vi "AudioTest, Audio Test Util, Manager.vi"(8 "error in (no error)":errorcluster, 11 "Config Folder":path=path "C:/MTE/Audio Test/Config") -> (0 "Error Out":errorcluster, 1 "Audio Test Result Path":path, 2 "Audio Test App Path":path, 3 "Meas":T1 {"Status" items=["LOG", "PASS", "FAIL", "ERROR"]})   [LabVIEW 2018]
uses:
  Common/Utils/Results/Result.Measurement Item.ctl
  Common/Utils/Results/Result.Measurement and Attribute Item Status.ctl
  Common/Utils/Cmd Exe/CmdConsole/CmdConsole.lvclass
  <vilib>/KATE/Files/File Utils.lvlib
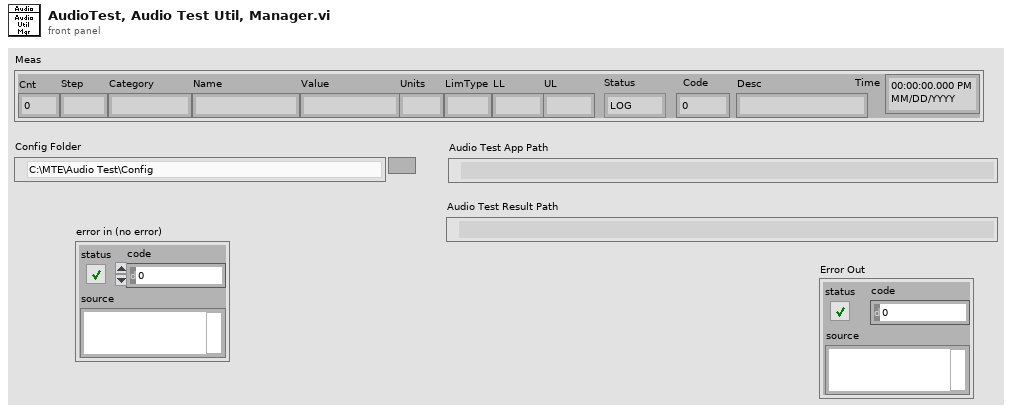
[diagram p1: front panel]
types:
  T1 = typedef "Result.Measurement Item.ctl" = cluster{"Cnt":i32, "Step":string, "Category":string, "Name":string, "Value":string, "Units":string, "LimType":string, "LL":string, "UL":string, "Status":T2, "Code":i32, "Desc":string, "Time":timestamp}
  T2 = typedef "Result.Measurement and Attribute Item Status.ctl" = i32
  T3 = enum32{"invalid app kind", "Development System", "Run Time System", "Student Edition", "Embedded LabVIEW", "Evaluation", "Custom"}
  T4 = cluster{"CmdConsole":refnum<class "CmdConsole.lvclass">, "OutDir":path, "Meas":T1}
  T5 = typedef "FunctTest.Result State.ctl" = enum32{"NoTest", "PASS", "FAIL"}
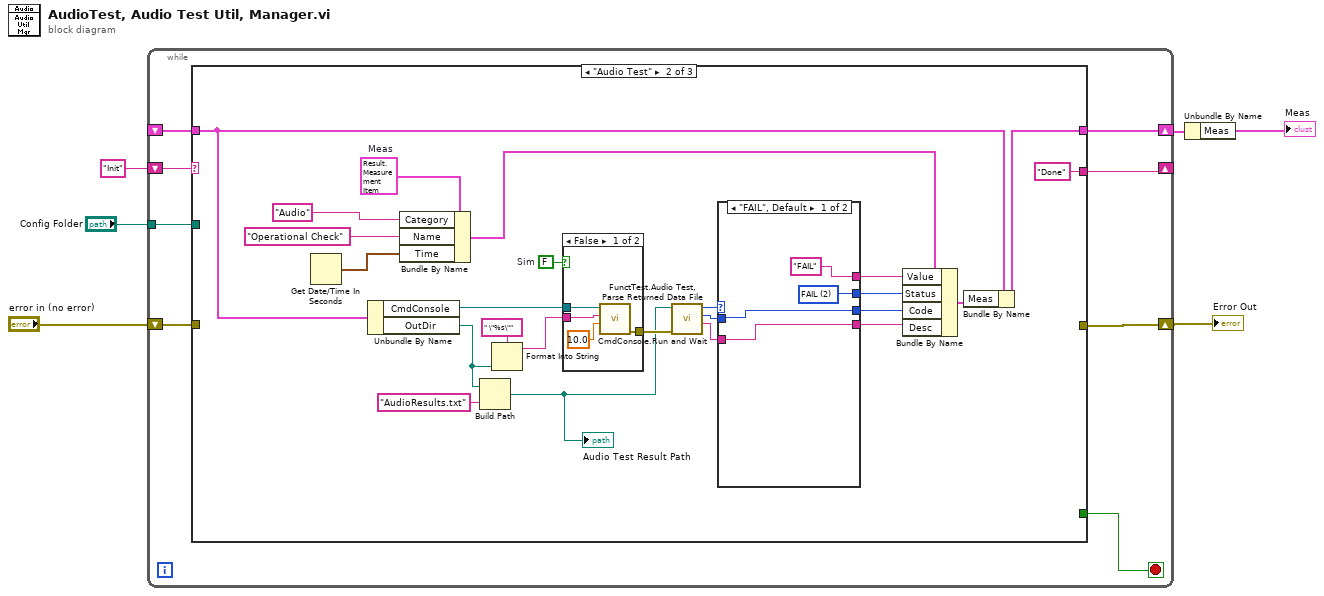
[diagram p0: block diagram]
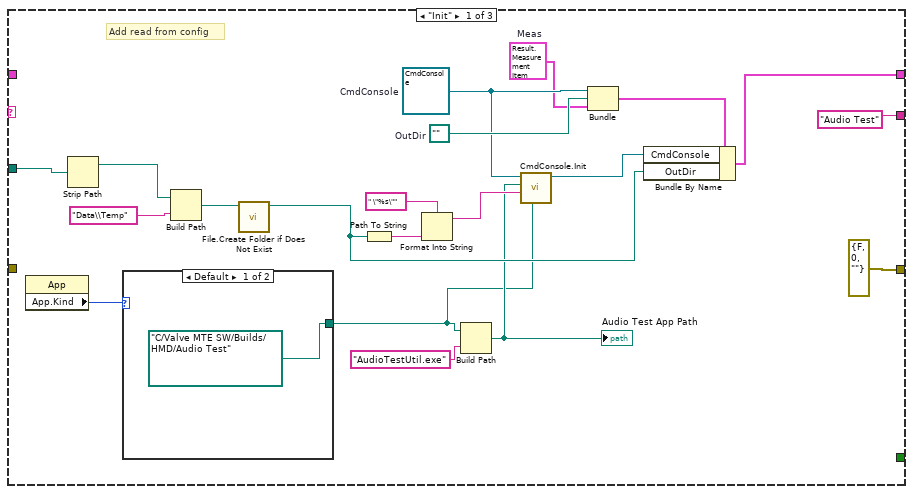
[diagram p2: hidden frame]
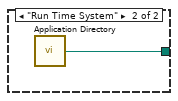
[diagram p3: hidden frame]
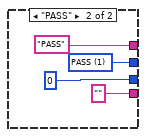
[diagram p4: hidden frame]
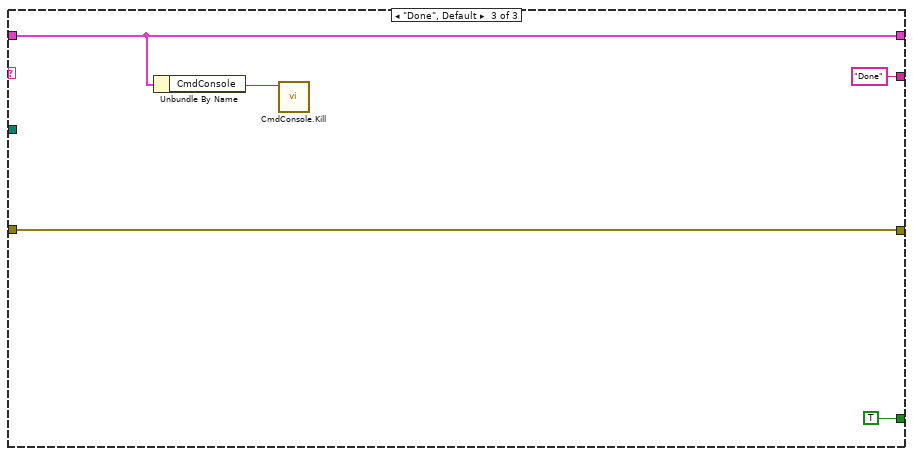
[diagram p6: hidden frame]
diagram:
  n1 = while {
    shift-right: [w13] -> w3
    shift-left: _ -> [w14]
    shift-right: [w11] -> w4
    shift-left: "error in (no error)" -> [w7]
    shift-right: [w9] -> _
    shift-left: "Init" -> [w10]
    tunnel: "Config Folder" -> [w8]
    stop <- w12 stop-if-true
    n2 = case shown="\"Audio Test\"" w10 {
      tunnel: w14 -> [_ w48 w74]
      tunnel: [w27 w47 w74] -> w13
      tunnel: [_ _ TRUE] -> w12
      tunnel: [errorcluster {"status"=FALSE, "code"=0, "source"=""} ("error constant") _ w75] -> w11
      tunnel: ["Audio Test" "Done" "Done"] -> w9
      tunnel: w8 -> [w22 _ _]
      tunnel: w7 -> [_ _ w75]
      frame "Init" {
        w16 = T1 {"Cnt"=0, "Step"="", "Category"="", "Name"="", "Value"="", "Units"="", "LimType"="", "LL"="", "UL"="", "Status"=0, "Code"=0, "Desc"="", "Time"=timestamp(0 s since 1904-01-01)}  # Meas
        w25 = refnum<class "CmdConsole.lvclass"> refnum  # CmdConsole
        w29 = path ""  # OutDir
        # "Add read from config"
        n3 = property class="App"() -> ("App.Kind"=w18:T3)  [unwired: 2 in, 2 out]
        n4 = Strip Path(path=w22) -> (stripped path=w21:path)  [unwired: 1 out]
        n5 = case shown="Default" w18 {
          tunnel: [path "C:/Valve MTE SW/Builds/HMD/Audio Test" w36] -> w15
          frame Default {
          }
          frame "Run Time System" {
            n6 = call <vilib>:"Application Directory.vi"() -> ("Application Directory"=w36:path)
          }
        }
        n7 = Build Path(base path=w21, name or relative path="Data\\Temp") -> (appended path=w20:path)
        n8 = call <vilib>:"File.Create Folder if Does Not Exist.vi"("Path"=w20) -> ("Dup Path"=w19:path)  [unwired: 8 in, 2 out]
        n9 = Path To String(path=w19) -> (string=w32:string)
        n10 = Format Into String(format string=" \"%s\"", w32) -> (resulting string=w30:string)  [unwired: 2 in, 1 out]
        n11 = Build Path(base path=w15, name or relative path="AudioTestUtil.exe") -> (appended path=w17:path)
        "Audio Test App Path" <- w17
        n12 = call "CmdConsole.Init.vi"("WorkingDir"=w15, "Args"=w30, "App"=w17, "CmdConsole in"=w25) -> ("CmdConsole out"=w26:refnum<class "CmdConsole.lvclass">)  [unwired: 6 in, 1 out]
        n13 = Bundle("CmdConsole"=w25, "OutDir"=w29, "Meas"=w16) -> (w28:T4)  [unwired: 1 in]
        n14 = Bundle By Name(cluster=w28, "CmdConsole"=w26, "OutDir"=w19) -> (w27:T4)
      }
      frame "Audio Test" {
        w46 = T1 {"Cnt"=0, "Step"="", "Category"="", "Name"="", "Value"="", "Units"="", "LimType"="", "LL"="", "UL"="", "Status"=0, "Code"=0, "Desc"="", "Time"=timestamp(0 s since 1904-01-01)}  # Meas
        w57 = FALSE  # Sim
        n15 = Get Date/Time In Seconds() -> (seconds since 1Jan1904=w37:timestamp)
        n16 = Unbundle By Name(w48) -> ("CmdConsole"=w59:refnum<class "CmdConsole.lvclass">, "OutDir"=w55:path)
        n17 = Bundle By Name(cluster=w46, "Category"="Audio", "Name"="Operational Check", "Time"=w37) -> (w43:T1)
        n18 = Build Path(base path=w55, name or relative path="AudioResults.txt") -> (appended path=w56:path)
        "Audio Test Result Path" <- w56
        n19 = Format Into String(format string=" \"%s\"", w55) -> (resulting string=w53:string)  [unwired: 2 in, 1 out]
        n20 = case shown="False" w57 {
          tunnel: w59 -> [w72 _]
          tunnel: [w70 _] -> w58
          tunnel: w53 -> [w69 _]
          frame False {
            n21 = call "CmdConsole.Run and Wait.vi"("Timeout(s)"=10.0 ("Duration"), "Args"=w69, "CmdConsole in"=w72) -> ("error out"=w70:errorcluster)  [unwired: 3 in, 5 out]
          }
          frame True {
          }
        }
        n22 = call "FunctTest.Audio Test, Parse Returned Data File.vi"("error in (no error)"=w58, "File Path"=w56) -> ("Desc"=w50:string, "Numeric"=w51:i32, "Result"=w52:T5)  [unwired: 7 in]
        n23 = case shown="\"FAIL\", Default" w52 {
          tunnel: w51 -> [w62 _]
          tunnel: w50 -> [w61 _]
          tunnel: [w62 0 ("AudioCode")] -> w41
          tunnel: ["FAIL" ("AudioResult") "PASS" ("AudioResult")] -> w40
          tunnel: [w64 w66] -> w39
          tunnel: [w61 ""] -> w38
          frame "FAIL", Default {
            w64 = T2 2 items=["LOG", "PASS", "FAIL", "ERROR"] ("Status")
          }
          frame "PASS" {
            w66 = T2 1 items=["LOG", "PASS", "FAIL", "ERROR"] ("Status")
          }
        }
        n24 = Bundle By Name(cluster=w43, "Value"=w40, "Status"=w39, "Code"=w41, "Desc"=w38) -> (w42:T1)
        n25 = Bundle By Name(cluster=w48, "Meas"=w42) -> (w47:T4)
      }
      frame "Done", Default {
        n26 = Unbundle By Name(w74) -> ("CmdConsole"=w73:refnum<class "CmdConsole.lvclass">)
        n27 = call "CmdConsole.Kill.vi"("CmdConsole in"=w73) -> ()  [unwired: 9 in, 2 out]
      }
    }
  }
  "Error Out" <- w4
  n28 = Unbundle By Name(w3) -> ("Meas"=→"Meas":T1)
